vi "SetImageBufferSize.vi"(8 "error in (no error)":errorcluster, 10 "max queue size (-1, unlimited)":i32, 11 "Camera_Prime95B in":refnum<class "Camera_Prime95B.lvclass">) -> (0 "error out":errorcluster, 3 "Camera_Prime95B out":refnum<class "Camera_Prime95B.lvclass">)   [LabVIEW 2020, in "Camera_Prime95B.lvlib" / "Camera_Prime95B.lvclass"]
uses:
  Camera_Prime95B.lvclass
  Camera_Prime95B.lvclass/Camera_Prime95B.ctl
  E:/Development/DevHardSoftware/MMicroscopyAF/Model/Real Hardware/Camera_Prime95B/Camera_Prime95B/Dependencies/PVCamNET.dll
  Dependencies/PVCamNET.dll
  HAL Layer/Component/Camera/Camera/Camera.lvclass
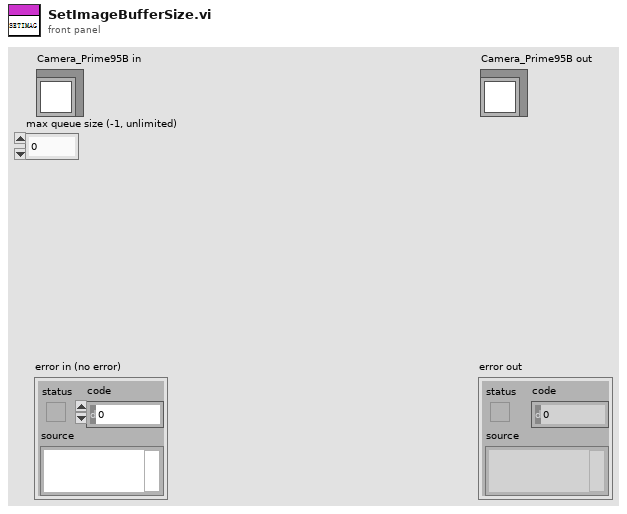
[diagram p1: front panel]
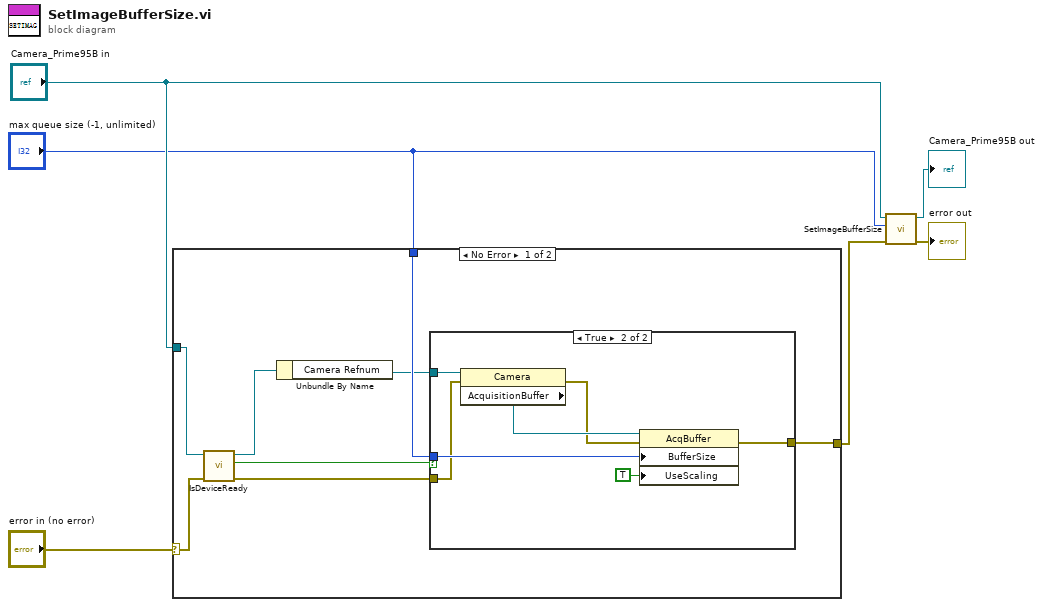
[diagram p0: block diagram]
diagram:
  n1 = case shown="No Error" "error in (no error)" {
    selector: "error in (no error)" -> [w12 w23]
    tunnel: [w13 w23] -> w1
    tunnel: "Camera_Prime95B in" -> [w11 _]
    tunnel: "max queue size (-1, unlimited)" -> [w14 _]
    frame No Error {
      n2 = call-dynamic "IsDeviceReady.vi"("error in (no error)"=w12, "Camera_Prime95B in"=w11) -> ("error out"=w10:errorcluster, "Ready?"=w9:bool, "Camera_Prime95B out"=w7:refnum<class "Camera_Prime95B.lvclass">)  [unwired: 7 in]
      n3 = Unbundle By Name(w7) -> ("Camera Refnum"=w8:refnum<k24>)
      n4 = case shown="True" w9 {
        tunnel: [w15 w22] -> w13
        tunnel: w14 -> [_ w19]
        tunnel: w10 -> [w15 w17]
        tunnel: w8 -> [_ w16]
        frame False {
        }
        frame True {
          n5 = property class="Camera"(reference=w16, error in=w17) -> (error out=w20:errorcluster, "AcquisitionBuffer"=w21:refnum<k24>)  [unwired: 1 out]
          n6 = property class="AcqBuffer"(reference=w21, error in=w20, "BufferSize"=w19, "UseScaling"=TRUE) -> (error out=w22:errorcluster)  [unwired: 1 out]
        }
      }
    }
    frame Error {
    }
  }
  n7 = call-parent "SetImageBufferSize.vi"("error in (no error)"=w1, "max queue size (-1, unlimited)"="max queue size (-1, unlimited)", "Camera in"="Camera_Prime95B in") -> ("error out"=→"error out":errorcluster, "Camera out"=→"Camera_Prime95B out":refnum<class "Camera_Prime95B.lvclass">)  [unwired: 7 in]
